vi "BuildFileSavePath.vi"(0 "Pixel Value":dbl, 2 "Base Path":path, 11 "DM Pixel":i32) -> (4 "DBL File Path":path, 8 "TXT File Path":path)   [LabVIEW 2016]
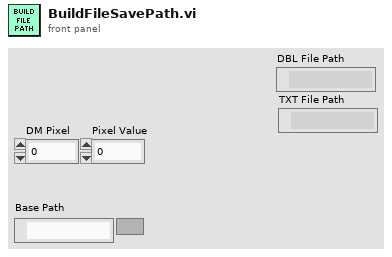
[diagram p1: front panel]
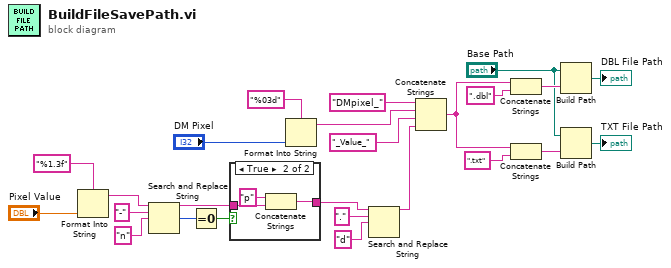
[diagram p0: block diagram]
diagram:
  n1 = Format Into String(format string="%1.3f", "Pixel Value") -> (resulting string=w20:string)  [unwired: 2 in, 1 out]
  n2 = Search and Replace String(input string=w20, search string="-", replace string="n" ("replace string (\"\")")) -> (result string=w15:string, number of replacements=w17:i32)  [unwired: 5 in, 2 out]
  n3 = Equal To 0?(x=w17) -> (x = 0?=w16:bool)
  n4 = case shown="True" w16 {
    tunnel: w15 -> [w26 w29]
    tunnel: [w26 w27] -> w12
    frame False {
    }
    frame True {
      n5 = Concatenate Strings("p" ("string"), w29) -> (w27:string)
    }
  }
  n6 = Format Into String(format string="%03d", "DM Pixel") -> (resulting string=w22:string)  [unwired: 2 in, 1 out]
  n7 = Search and Replace String(input string=w12, search string=".", replace string="d" ("replace string (\"\")")) -> (result string=w11:string)  [unwired: 5 in, 3 out]
  n8 = Concatenate Strings("DMpixel_", w22, "_Value_", w11) -> (w8:string)
  n9 = Concatenate Strings(w8, ".dbl" ("string")) -> (w5:string)
  n10 = Concatenate Strings(w8, ".txt" ("string")) -> (w4:string)
  n11 = Build Path(base path="Base Path", name or relative path=w5) -> (appended path=→"DBL File Path":path)
  n12 = Build Path(base path="Base Path", name or relative path=w4) -> (appended path=→"TXT File Path":path)
